vi "maze_v6.vi"   [LabVIEW 2012]
uses:
  <vilib>/NXT/Subs/MotorOutput.ctl
  <vilib>/NXT/Block Support/NXT_InputPort.ctl
  <vilib>/NXT/Dual Mode Library/Motors/MotorBrake.vi
  <vilib>/NXT/Dual Mode Library/Motors/MotorOn.vi
  <vilib>/NXT/Dual Mode Library/Motors/MotorReverse.vi
  <vilib>/NXT/Dual Mode Library/prims/addArrayElements_int.vi
  <vilib>/NXT/Dual Mode Library/Waits/Wait_Num(msec).vi
  <vilib>/NXT/Dual Mode Library/Sound/Tone.vi
types:
  T1 = typedef "MotorOutput.ctl" = u8
  T2 = typedef "LVHSConnector.ctl" = cluster{"Hardware":string, "Flattened String":string}
  T3 = typedef "NXT_InputPort.ctl" = u8
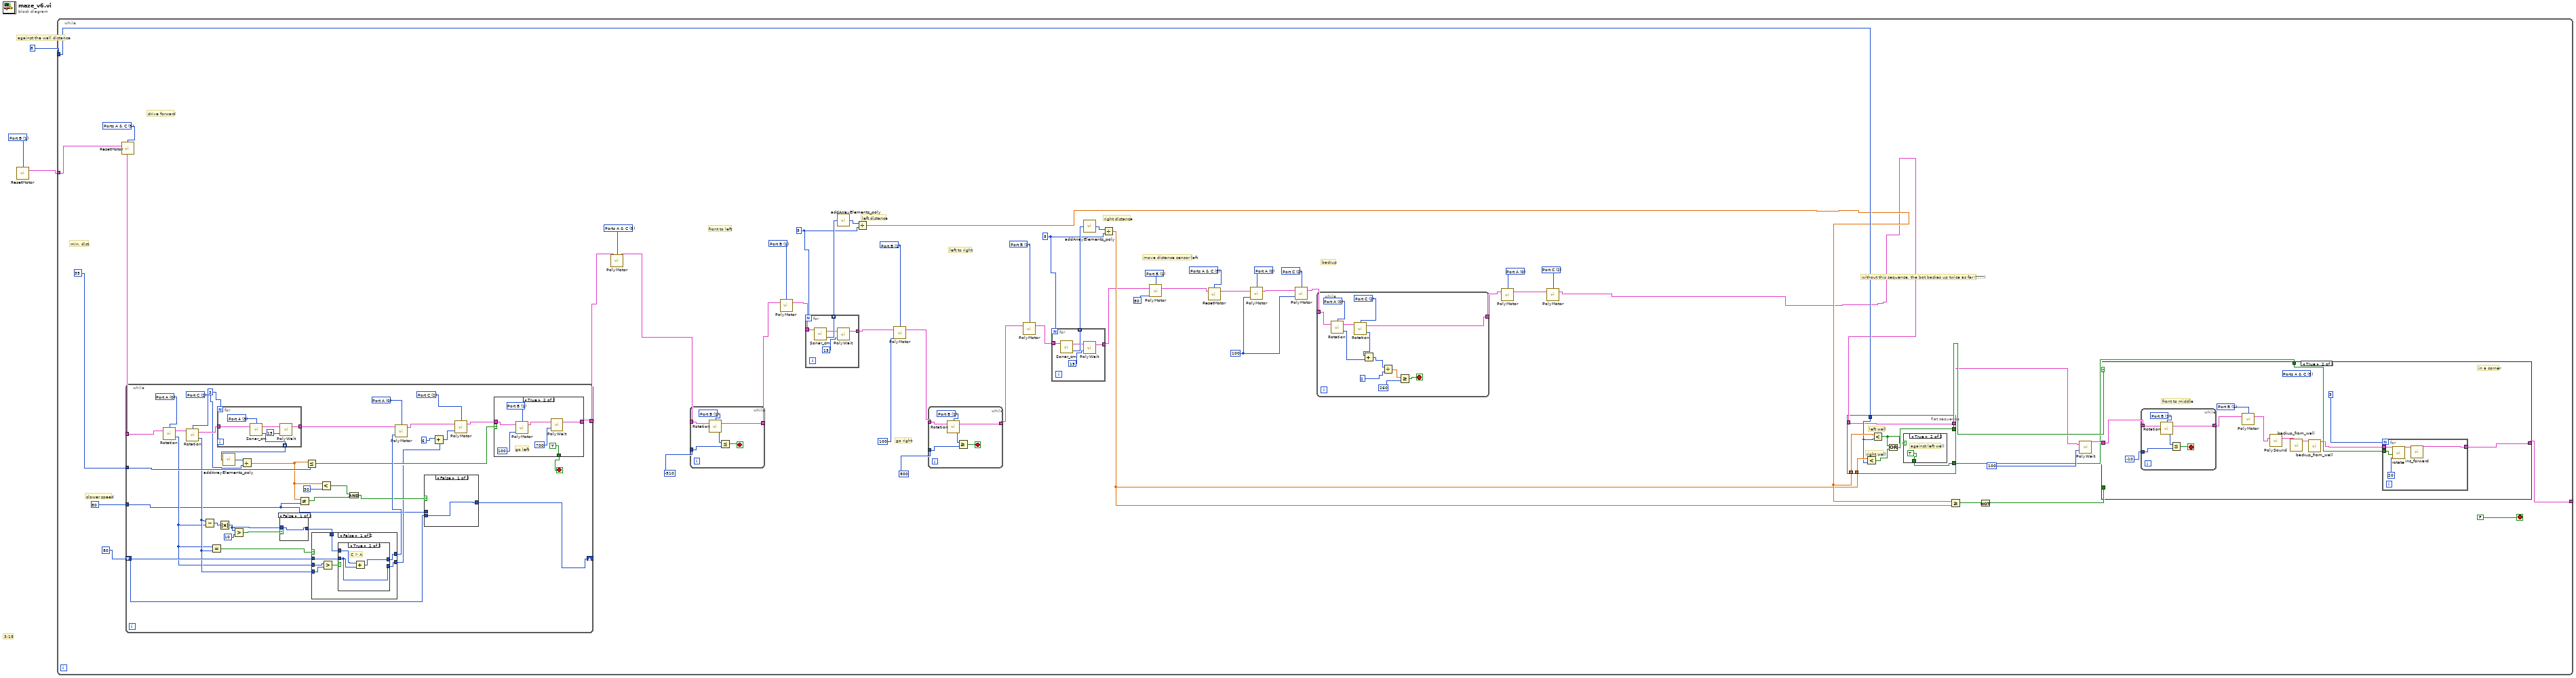
[diagram p0: block diagram]
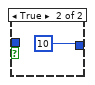
[diagram p2: hidden frame]
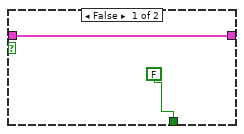
[diagram p4: hidden frame]
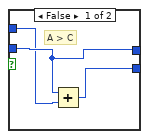
[diagram p5: hidden frame]
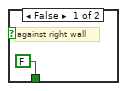
[diagram p7: hidden frame]
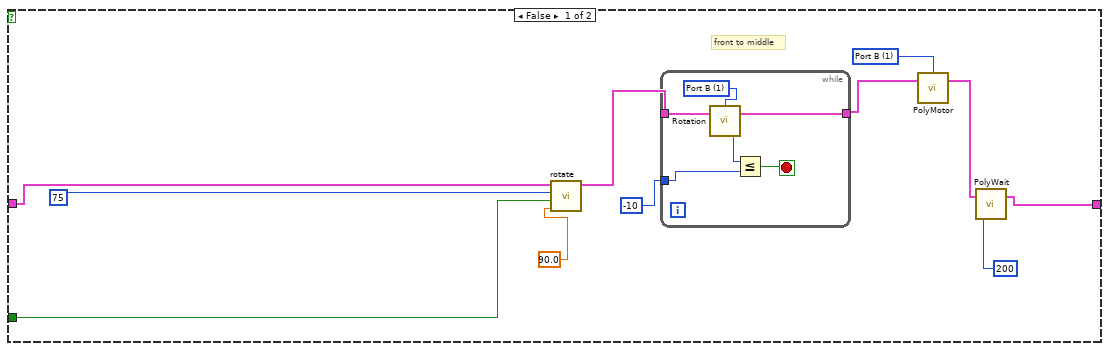
[diagram p8: hidden frame]
diagram:
  w3 = T1 1 items=["Port A"=0, "Port B"=1, "Port C"=2, "Ports A & B"=4, "Ports A & C"=5, "Ports B & C"=6, "All Ports"=3] ("Output Port (All Ports)")
  # "3:15"
  # "against the wall distance"
  n1 = call <vilib>:"ResetMotor.vi"("Port (All Ports)"=w3) -> ("NXT"=w1:T2)  [unwired: 3 in]
  n2 = while {
    tunnel: u16 8 ("power") -> [w53]
    tunnel: [w50] -> _
    tunnel: w1 -> [w42]
    stop <- FALSE stop-if-true
    w8 = T1 1 items=["Port A"=0, "Port B"=1, "Port C"=2, "Ports A & B"=4, "Ports A & C"=5, "Ports B & C"=6, "All Ports"=3] ("Output Port (All Ports)")
    w13 = T1 2 items=["Port A"=0, "Port B"=1, "Port C"=2, "Ports A & B"=4, "Ports A & C"=5, "Ports B & C"=6, "All Ports"=3] ("Output Port (All Ports)")
    w11 = T1 0 items=["Port A"=0, "Port B"=1, "Port C"=2, "Ports A & B"=4, "Ports A & C"=5, "Ports B & C"=6, "All Ports"=3] ("Output Port (All Ports)")
    w15 = 100
    w17 = T1 2 items=["Port A"=0, "Port B"=1, "Port C"=2, "Ports A & B"=4, "Ports A & C"=5, "Ports B & C"=6, "All Ports"=3] ("Output Port (All Ports)")
    w19 = T1 0 items=["Port A"=0, "Port B"=1, "Port C"=2, "Ports A & B"=4, "Ports A & C"=5, "Ports B & C"=6, "All Ports"=3] ("Output Port (All Ports)")
    w20 = T1 5 items=["Port A"=0, "Port B"=1, "Port C"=2, "Ports A & B"=4, "Ports A & C"=5, "Ports B & C"=6, "All Ports"=3] ("Output Port (All Ports)")
    w25 = 5
    w28 = 5
    w35 = T1 1 items=["Port A"=0, "Port B"=1, "Port C"=2, "Ports A & B"=4, "Ports A & C"=5, "Ports B & C"=6, "All Ports"=3] ("Output Port (All Ports)")
    w36 = T1 1 items=["Port A"=0, "Port B"=1, "Port C"=2, "Ports A & B"=4, "Ports A & C"=5, "Ports B & C"=6, "All Ports"=3] ("Output Port (All Ports)")
    w40 = T1 1 items=["Port A"=0, "Port B"=1, "Port C"=2, "Ports A & B"=4, "Ports A & C"=5, "Ports B & C"=6, "All Ports"=3] ("Output Port (All Ports)")
    w49 = T1 5 items=["Port A"=0, "Port B"=1, "Port C"=2, "Ports A & B"=4, "Ports A & C"=5, "Ports B & C"=6, "All Ports"=3] ("Output Port (All Ports)")
    w47 = T1 5 items=["Port A"=0, "Port B"=1, "Port C"=2, "Ports A & B"=4, "Ports A & C"=5, "Ports B & C"=6, "All Ports"=3] ("Output Port (All Ports)")
    # "move distance sensor left"
    # "backup"
    # "right distance"
    # "left distance"
    # "go right"
    # "left to right"
    # "front to left"
    # "drive forward"
    # "min. dist."
    # "slower speed"
    # "without this sequence, the bot backes up twice as far (????)"
    n3 = call <vilib>:"ResetMotor.vi"("NXT"=w42, "Port (All Ports)"=w47) -> ("NXT"=w48:T2)  [unwired: 2 in]
    n4 = while {
      tunnel: w48 -> [w129]
      tunnel: [w117] -> w46
      tunnel: 35 -> [w119]
      shift-right: [w109] -> _
      shift-left: 80 -> [w108]
      tunnel: 80 -> [w93]
      stop <- w114 stop-if-true
      w94 = 3
      w122 = T1 2 items=["Port A"=0, "Port B"=1, "Port C"=2, "Ports A & B"=4, "Ports A & C"=5, "Ports B & C"=6, "All Ports"=3] ("Output Port (All Ports)")
      w123 = T1 0 items=["Port A"=0, "Port B"=1, "Port C"=2, "Ports A & B"=4, "Ports A & C"=5, "Ports B & C"=6, "All Ports"=3] ("Output Port (All Ports)")
      w124 = T1 2 items=["Port A"=0, "Port B"=1, "Port C"=2, "Ports A & B"=4, "Ports A & C"=5, "Ports B & C"=6, "All Ports"=3] ("Output Port (All Ports)")
      w125 = T1 0 items=["Port A"=0, "Port B"=1, "Port C"=2, "Ports A & B"=4, "Ports A & C"=5, "Ports B & C"=6, "All Ports"=3] ("Output Port (All Ports)")
      n5 = call <vilib>:"Rotation.vi"("NXT"=w129, "Port (Port A)"=w123) -> ("Angle of Rotation"=w106:i32, "NXT"=w128:T2)  [unwired: 1 in]
      n6 = call <vilib>:"Rotation.vi"("NXT"=w128, "Port (Port A)"=w122) -> ("Angle of Rotation"=w107:i32, "NXT"=w127:T2)  [unwired: 1 in]
      n7 = Subtract(x=w107, y=w106) -> (x-y=w105:i32)
      n8 = Equal?(x=w106, y=w107) -> (x = y?=w121:bool)
      n9 = for {
        N: w94 -> [_]
        tunnel: w127 -> [w134]
        tunnel: [w132] -> w120
        tunnel: [w133] -> w97 mode=indexing
        w135 = T3 3 items=["Port 1", "Port 2", "Port 3", "Port 4"] ("Port (Port 4)")
        n10 = call <vilib>:"Sonar_cm.vi"("NXT"=w134, "Port (Port 4)"=w135) -> ("Distance (cm)"=w133:i16, "NXT"=w131:T2)  [unwired: 1 in]
        n11 = call-poly <vilib>:"PolyWait.vi"("Time (100 msec)"=15, "NXT"=w131) -> ("NXT"=w132:T2)  [unwired: 2 in]
      }
      n12 = Absolute Value(x=w105) -> (abs(x)=w102:i32)
      n13 = call-poly <vilib>:"addArrayElements_poly.vi"("Numeric Array"=w97) -> ("Sum"=w96:i32)
      n14 = Greater?(x=w102, y=10) -> (0:w103:bool)
      n15 = Divide(x=w96, y=w94) -> (x/y=w95:dbl)
      n16 = case shown="False" w103 {
        tunnel: [w136 10] -> w101
        tunnel: w102 -> [w136 _]
        frame False {
        }
        frame True {
        }
      }
      n17 = Not Equal?(x=w95, y=w93) -> (x != y?=w111:bool)
      n18 = Less Or Equal?(x=w95, y=w119) -> (x <= y?=w115:bool)
      n19 = case shown="False" w121 {
        tunnel: [w153 w162] -> w118
        tunnel: w108 -> [w154 w162]
        tunnel: [w152 w162] -> w99
        tunnel: w107 -> [w151 _]
        tunnel: w106 -> [w150 _]
        tunnel: w101 -> [w149 _]
        frame False {
          n20 = Greater?(x=w150, y=w151) -> (0:w155:bool)
          n21 = case shown="True" w155 {
            tunnel: w154 -> [w157 w161]
            tunnel: [w157 w159] -> w153
            tunnel: [w158 w161] -> w152
            tunnel: w149 -> [w156 w160]
            frame False {
              # "A > C"
              n22 = Add(x=w157, y=w156) -> (x+y=w158:i32)
            }
            frame True {
              # "C > A"
              n23 = Add(x=w160, y=w161) -> (x+y=w159:i32)
            }
          }
        }
        frame True {
        }
      }
      n24 = Less?(x=w95, y=30) -> (x < y?=w112:bool)
      n25 = And(x=w112, y=w111) -> (x .and. y?=w110:bool)
      n26 = call-poly <vilib>:"PolyMotor.vi"("Power (75)"=w118, "NXT"=w120, "Output Port (All Ports)"=w125) -> ("NXT"=w126:T2)  [unwired: 1 in]
      n27 = case shown="False" w110 {
        tunnel: [w138 w139] -> w109
        tunnel: w108 -> [w138 _]
        tunnel: w93 -> [_ w139]
        frame False {
        }
        frame True {
        }
      }
      n28 = Add(x=6, y=w99) -> (x+y=w98:i32)
      n29 = call-poly <vilib>:"PolyMotor.vi"("Power (75)"=w98, "NXT"=w126, "Output Port (All Ports)"=w124) -> ("NXT"=w116:T2)  [unwired: 1 in]
      n30 = case shown="True" w115 {
        tunnel: [w140 w148] -> w117
        tunnel: w116 -> [w140 w143]
        tunnel: [FALSE TRUE] -> w114
        frame False {
        }
        frame True {
          w145 = T1 1 items=["Port A"=0, "Port B"=1, "Port C"=2, "Ports A & B"=4, "Ports A & C"=5, "Ports B & C"=6, "All Ports"=3] ("Output Port (All Ports)")
          # "go left"
          n31 = call-poly <vilib>:"PolyMotor.vi"("Power (75)"=100, "NXT"=w143, "Output Port (All Ports)"=w145) -> ("NXT"=w142:T2)  [unwired: 1 in]
          n32 = call-poly <vilib>:"PolyWait.vi"("Time (100 msec)"=700, "NXT"=w142) -> ("NXT"=w148:T2)  [unwired: 2 in]
        }
      }
    }
    n33 = call-poly <vilib>:"PolyMotor.vi"("NXT"=w46, "Port (All Ports)"=w49) -> ("NXT"=w21:T2)  [unwired: 2 in]
    n34 = while {
      tunnel: -510 -> [w91]
      tunnel: w21 -> [w89]
      tunnel: [w88] -> w39
      stop <- w87 stop-if-true
      w90 = T1 1 items=["Port A"=0, "Port B"=1, "Port C"=2, "Ports A & B"=4, "Ports A & C"=5, "Ports B & C"=6, "All Ports"=3] ("Output Port (All Ports)")
      n35 = call <vilib>:"Rotation.vi"("NXT"=w89, "Port (Port A)"=w90) -> ("Angle of Rotation"=w92:i32, "NXT"=w88:T2)  [unwired: 1 in]
      n36 = Less Or Equal?(x=w92, y=w91) -> (x <= y?=w87:bool)
    }
    n37 = call-poly <vilib>:"PolyMotor.vi"("NXT"=w39, "Port (All Ports)"=w40) -> ("NXT"=w32:T2)  [unwired: 2 in]
    n38 = for {
      N: w28 -> [_]
      tunnel: w32 -> [w79]
      tunnel: [w80] -> w30 mode=indexing
      tunnel: [w77] -> w31
      n39 = call <vilib>:"Sonar_cm.vi"("NXT"=w79) -> ("Distance (cm)"=w80:i16, "NXT"=w78:T2)  [unwired: 2 in]
      n40 = call-poly <vilib>:"PolyWait.vi"("Time (100 msec)"=15, "NXT"=w78) -> ("NXT"=w77:T2)  [unwired: 2 in]
    }
    n41 = call-poly <vilib>:"addArrayElements_poly.vi"("Numeric Array"=w30) -> ("Sum"=w29:i32)
    n42 = Divide(x=w29, y=w28) -> (x/y=w23:dbl)
    n43 = call-poly <vilib>:"PolyMotor.vi"("Power (75)"=100, "NXT"=w31, "Output Port (All Ports)"=w36) -> ("NXT"=w37:T2)  [unwired: 1 in]
    n44 = while {
      tunnel: 800 -> [w85]
      tunnel: w37 -> [w83]
      tunnel: [w82] -> w34
      stop <- w81 stop-if-true
      w84 = T1 1 items=["Port A"=0, "Port B"=1, "Port C"=2, "Ports A & B"=4, "Ports A & C"=5, "Ports B & C"=6, "All Ports"=3] ("Output Port (All Ports)")
      n45 = call <vilib>:"Rotation.vi"("NXT"=w83, "Port (Port A)"=w84) -> ("Angle of Rotation"=w86:i32, "NXT"=w82:T2)  [unwired: 1 in]
      n46 = Greater Or Equal?(x=w86, y=w85) -> (x >= y?=w81:bool)
    }
    n47 = call-poly <vilib>:"PolyMotor.vi"("NXT"=w34, "Port (All Ports)"=w35) -> ("NXT"=w24:T2)  [unwired: 2 in]
    n48 = for {
      N: w25 -> [_]
      tunnel: w24 -> [w74]
      tunnel: [w75] -> w27 mode=indexing
      tunnel: [w72] -> w7
      n49 = call <vilib>:"Sonar_cm.vi"("NXT"=w74) -> ("Distance (cm)"=w75:i16, "NXT"=w73:T2)  [unwired: 2 in]
      n50 = call-poly <vilib>:"PolyWait.vi"("Time (100 msec)"=15, "NXT"=w73) -> ("NXT"=w72:T2)  [unwired: 2 in]
    }
    n51 = call-poly <vilib>:"addArrayElements_poly.vi"("Numeric Array"=w27) -> ("Sum"=w26:i32)
    n52 = Divide(x=w26, y=w25) -> (x/y=w22:dbl)
    n53 = call-poly <vilib>:"PolyMotor.vi"("Power (75)"=80, "NXT"=w7, "Output Port (All Ports)"=w8) -> ("NXT"=w6:T2)  [unwired: 1 in]
    n54 = call <vilib>:"ResetMotor.vi"("NXT"=w6, "Port (All Ports)"=w20) -> ("NXT"=w14:T2)  [unwired: 2 in]
    n55 = call-poly <vilib>:"PolyMotor.vi"("Power (75)"=w15, "NXT"=w14, "Output Port (All Ports)"=w19) -> ("NXT"=w18:T2)  [unwired: 1 in]
    n56 = call-poly <vilib>:"PolyMotor.vi"("Power (75)"=w15, "NXT"=w18, "Output Port (All Ports)"=w17) -> ("NXT"=w16:T2)  [unwired: 1 in]
    n57 = while {
      tunnel: w16 -> [w68]
      tunnel: [w59] -> w10
      stop <- w61 stop-if-true
      w67 = T1 2 items=["Port A"=0, "Port B"=1, "Port C"=2, "Ports A & B"=4, "Ports A & C"=5, "Ports B & C"=6, "All Ports"=3] ("Output Port (All Ports)")
      w69 = T1 0 items=["Port A"=0, "Port B"=1, "Port C"=2, "Ports A & B"=4, "Ports A & C"=5, "Ports B & C"=6, "All Ports"=3] ("Output Port (All Ports)")
      n58 = call <vilib>:"Rotation.vi"("NXT"=w68, "Port (Port A)"=w69) -> ("Angle of Rotation"=w64:i32, "NXT"=w70:T2)  [unwired: 1 in]
      n59 = call <vilib>:"Rotation.vi"("NXT"=w70, "Port (Port A)"=w67) -> ("Angle of Rotation"=w63:i32, "NXT"=w59:T2)  [unwired: 1 in]
      n60 = Add(x=w63, y=w64) -> (x+y=w65:i32)
      n61 = Divide(x=w65, y=2) -> (x/y=w60:dbl)
      n62 = Greater Or Equal?(x=w60, y=260) -> (x >= y?=w61:bool)
    }
    n63 = call-poly <vilib>:"PolyMotor.vi"("NXT"=w10, "Port (All Ports)"=w11) -> ("NXT"=w12:T2)  [unwired: 2 in]
    n64 = call-poly <vilib>:"PolyMotor.vi"("NXT"=w12, "Port (All Ports)"=w13) -> ("NXT"=w5:T2)  [unwired: 2 in]
    n65 = flat-sequence {
      tunnel: [w163] -> w4
      tunnel: w22 -> [w170]
      tunnel: w53 -> [w168]
      tunnel: w23 -> [w169]
      tunnel: [w166] -> w52
      tunnel: [w164] -> w51
      tunnel: w5 -> [w163]
      frame #0 {
        # "left wall"
        # "right wall"
        n66 = Less?(x=w170, y=w168) -> (x < y?=w167:bool)
        n67 = Less?(x=w169, y=w168) -> (x < y?=w165:bool)
        n68 = Or(x=w165, y=w167) -> (x .or. y?=w166:bool)
        n69 = case shown="True" w165 {
          tunnel: [FALSE TRUE] -> w164
          frame False {
            # "against right wall"
          }
          frame True {
            # "against left wall"
          }
        }
      }
    }
    n70 = Greater Or Equal?(x=w23, y=w22) -> (x >= y?=w57:bool)
    n71 = Not(x=w57) -> (.not. x?=w56:bool)
    n72 = call-poly <vilib>:"PolyWait.vi"("Time (100 msec)"=u16 100 ("power"), "NXT"=w4) -> ("NXT"=w55:T2)  [unwired: 2 in]
    n73 = case shown="True" w52 {
      tunnel: w51 -> [_ w197]
      tunnel: w55 -> [w179 w191]
      tunnel: [w178 w195] -> w50
      tunnel: w56 -> [w182 _]
      frame False {
        w176 = T1 1 items=["Port A"=0, "Port B"=1, "Port C"=2, "Ports A & B"=4, "Ports A & C"=5, "Ports B & C"=6, "All Ports"=3] ("Output Port (All Ports)")
        # "front to middle"
        n74 = call "rotate.vi"("degrees to  rotate"=90.0, "right(T)/left(F)"=w182, "power"=u16 75, "NXT 2"=w179) -> ("NXT"=w174:T2)  [unwired: 7 in]
        n75 = while {
          tunnel: -10 -> [w188]
          tunnel: [w186] -> w175
          tunnel: w174 -> [w184]
          stop <- w185 stop-if-true
          w187 = T1 1 items=["Port A"=0, "Port B"=1, "Port C"=2, "Ports A & B"=4, "Ports A & C"=5, "Ports B & C"=6, "All Ports"=3] ("Output Port (All Ports)")
          n76 = call <vilib>:"Rotation.vi"("NXT"=w184, "Port (Port A)"=w187) -> ("Angle of Rotation"=w189:i32, "NXT"=w186:T2)  [unwired: 1 in]
          n77 = Less Or Equal?(x=w189, y=w188) -> (x <= y?=w185:bool)
        }
        n78 = call-poly <vilib>:"PolyMotor.vi"("NXT"=w175, "Port (All Ports)"=w176) -> ("NXT"=w173:T2)  [unwired: 2 in]
        n79 = call-poly <vilib>:"PolyWait.vi"("Time (100 msec)"=i16 200 ("degrees to  rotate"), "NXT"=w173) -> ("NXT"=w178:T2)  [unwired: 2 in]
      }
      frame True {
        w193 = T1 1 items=["Port A"=0, "Port B"=1, "Port C"=2, "Ports A & B"=4, "Ports A & C"=5, "Ports B & C"=6, "All Ports"=3] ("Output Port (All Ports)")
        (unwired) T1 5 items=["Port A"=0, "Port B"=1, "Port C"=2, "Ports A & B"=4, "Ports A & C"=5, "Ports B & C"=6, "All Ports"=3] ("Output Port (All Ports)")
        # "front to middle"
        # "in a corner"
        n80 = while {
          tunnel: -10 -> [w205]
          tunnel: [w203] -> w192
          tunnel: w191 -> [w201]
          stop <- w202 stop-if-true
          w204 = T1 1 items=["Port A"=0, "Port B"=1, "Port C"=2, "Ports A & B"=4, "Ports A & C"=5, "Ports B & C"=6, "All Ports"=3] ("Output Port (All Ports)")
          n81 = call <vilib>:"Rotation.vi"("NXT"=w201, "Port (Port A)"=w204) -> ("Angle of Rotation"=w206:i32, "NXT"=w203:T2)  [unwired: 1 in]
          n82 = Less Or Equal?(x=w206, y=w205) -> (x <= y?=w202:bool)
        }
        n83 = call-poly <vilib>:"PolyMotor.vi"("NXT"=w192, "Port (All Ports)"=w193) -> ("NXT"=w190:T2)  [unwired: 2 in]
        n84 = call-poly <vilib>:"PolySound.vi"("NXT"=w190) -> ("NXT"=w200:T2)  [unwired: 3 in]
        n85 = call "backup_from_wall.vi"("NXT"=w200) -> ("NXT2"=w199:T2)  [unwired: 10 in]
        n86 = call "backup_from_wall.vi"("NXT"=w199) -> ("NXT2"=w196:T2)  [unwired: 10 in]
        n87 = for {
          N: u16 3 ("power") -> [_]
          tunnel: w197 -> [w210]
          tunnel: w196 -> [w209]
          tunnel: [w207] -> w195
          n88 = call "rotate.vi"("degrees to  rotate"=u16 20 ("power"), "right(T)/left(F)"=w210, "NXT 2"=w209) -> ("NXT"=w208:T2)  [unwired: 8 in]
          n89 = call "inc_forward.vi"("NXT"=w208) -> ("NXT2"=w207:T2)  [unwired: 10 in]
        }
      }
    }
  }
